vi "Write HWND.vi"(8 "error in (no error)":errorcluster, 10 "HWND":i32, 11 "Container base in":refnum<class "Container base.lvclass">) -> (0 "error out":errorcluster, 3 "Container base out":refnum<class "Container base.lvclass">)   [LabVIEW 2019, in "Container base.lvclass"]
doc: "Write HWND."
uses:
  Container base.lvclass
  Container base.lvclass/Container base.ctl
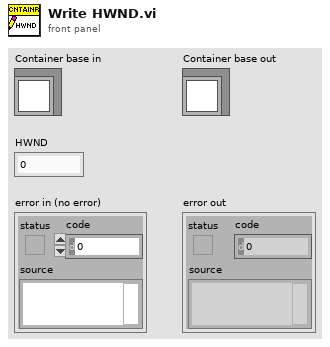
[diagram p1: front panel]
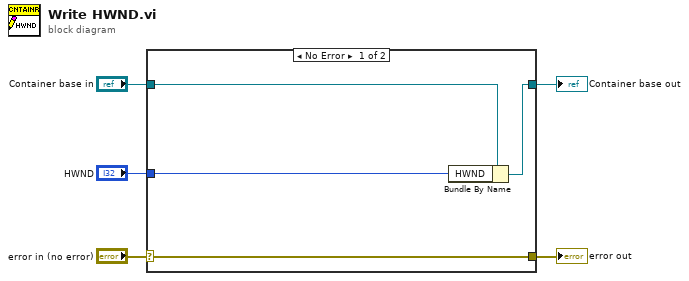
[diagram p0: block diagram]
diagram:
  n1 = case shown="No Error" "error in (no error)" {
    selector: "error in (no error)" -> [w9 w10]
    tunnel: [w9 w10] -> w4
    tunnel: [w7 w11] -> w2
    tunnel: "Container base in" -> [w8 w11]
    tunnel: "HWND" -> [w6 _]
    frame No Error {
      n2 = Bundle By Name(cluster=w8, "HWND"=w6) -> (w7:refnum<class "Container base.lvclass">)
    }
    frame Error {
    }
  }
  "error out" <- w4
  "Container base out" <- w2
